vi "StablizeDriving.vi"(10 "AngleSetpoints":dbl[](array[numeric]), 11 "Enable":bool) -> (3 "NewAngles":dbl[](array[numeric]))   [LabVIEW 2019]
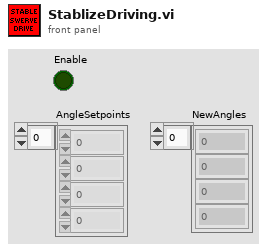
[diagram p1: front panel]
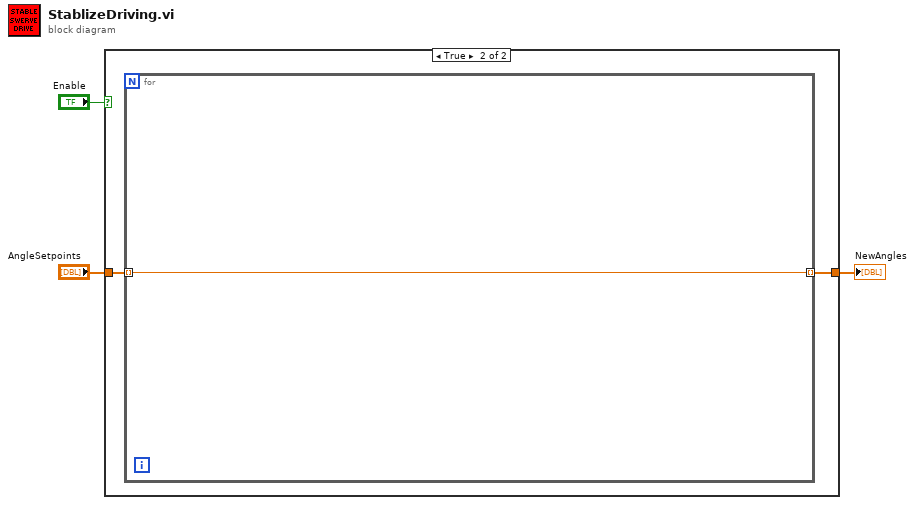
[diagram p0: block diagram]
diagram:
  n1 = case shown="True" "Enable" {
    tunnel: "AngleSetpoints" -> [w4 w6]
    tunnel: [w4 w5] -> w1
    frame False {
    }
    frame True {
      n2 = for {
        tunnel: w6 -> [w7] mode=indexing
        tunnel: [w7] -> w5 mode=indexing
      }
    }
  }
  "NewAngles" <- w1
